vi "MICSD Zarlink Telemetry.vi"(6 "Transceive Delay mS":dbl=200.0 min=0.0 max=10000.0 step=1.0, 7 "EXID":u32=16773121 step=1 format="%.0x", 8 "Parameters":string, 9 "CP_DATA IN":u8[](array[numeric]), 10 "Function":T3(ring)=enum."Downlink Only", 11 "Command":T2) -> (0 "Data":string, 1 "CP_DATA OUT":u8[](array[numeric]), 2 "Response Code":string, 3 "Response Token":string, 4 "tChecksum Valid":bool, 5 "bChecksum Valid":bool)   [LabVIEW 2010]
uses:
  Zarlink Telemetry v9_0/Telemetry/Typedef Command List.ctl
  <vilib>/Utility/file.llb/Write To Spreadsheet File (string).vi
panel:
  out "Status Flags":T1
  in  "RF_Channel":u8=3
  in  "VISA Resource Name":refnum<visa-resource-name>="COM3"
  in  "Target MICS ID":u32=1048576 step=1 format="%.0x"
  out "error out":errorcluster
  in  "error in (no error)":errorcluster
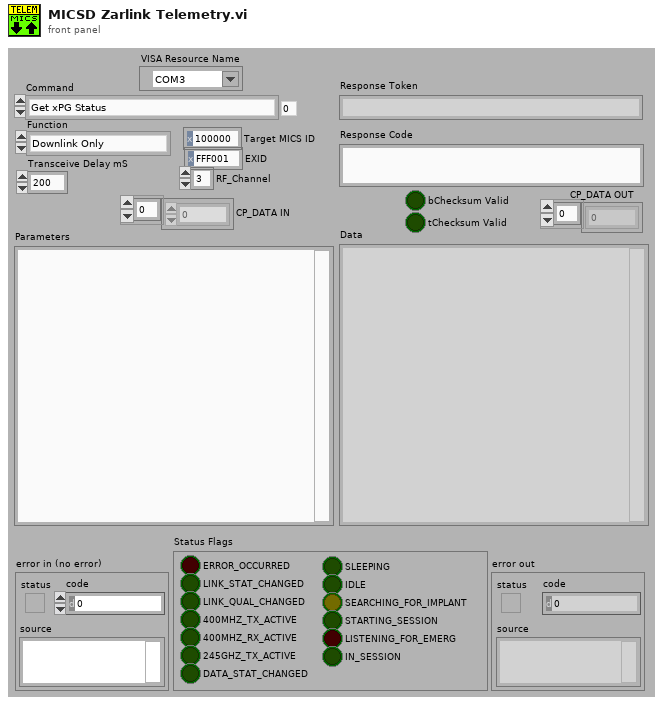
[diagram p1: front panel]
types:
  T1 = cluster{"ERROR_OCCURRED":bool, "LINK_STAT_CHANGED":bool, "LINK_QUAL_CHANGED":bool, "400MHZ_TX_ACTIVE":bool, "400MHZ_RX_ACTIVE":bool, "245GHZ_TX_ACTIVE":bool, "DATA_STAT_CHANGED":bool, "SLEEPING":bool, "IDLE":bool, "SEARCHING_FOR_IMPLANT":bool, "STARTING_SESSION":bool, "LISTENING_FOR_EMERG":bool, "IN_SESSION":bool}
  T2 = typedef "Typedef Command List.ctl" = enum16{"Get xPG Status", "xPG Stimulation", "Select Program", "Increment Program Amplitude", "Decrement Program Amplitude", "Get PoP Constants", "Get PPC Constants", "Get Program Names", "Set Pulse Amplitude", "Increment Pulse Amplitude", "Decrement Pulse Amplitude", "Get Pulse Widths", "Set Pulse Widths", "Increment Pulse Width", "Decrement Pulse Width", "Get Program Frequency", "Set Program Frequency", "Increment Program Frequency", "Decrement Program Frequency", "<reserved 1>", "Charging Control", "Get xPG Identity", "Set xPG Identity", "Restore Program Defaults", "Get Program Definition", "Set Program Definition", "Get Program Constants", "Set Program Constants", "Get Configurable Device Parameters", "Set Configurable Device Parameters", "Get Pulse Constants", "Set Pulse Constants", "Get Lead Limits", "Set Lead Limits", "Get Channel Calibrations", "Set Channel Calibrations", "<reserved 2>", "<reserved 3>", "<reserved 4>", "<reserved 5>", "<reserved 6>", "<reserved 7>", "Get Stim Asic HV Calibrations", "Set Stim Asic HV Calibrations", "<reserved 8>", "<reserved 9>", "Get CP Data", "Set CP Data", "Clear Log", "Read Log", "Append Log", "Get Patient Program Runtime", "Set Patient Program Runtime", "Impedance Measurement", "Enter Storage Mode", "Echo Short", "Echo Long", "Get General Calibration", "Set General Calibration", "Get Trim List", "Set Trim List", "Get Counter", "Set Counter", "Get Test Stimulation", "Set Test Stimulation", "Get Titration Stimulation", "Set Titration Stimulation", "Get Ramp Time", "Set Ramp Time", "Get VBAT", "Set Software Description Block", "Get Software Description Block", "Write Memory", "Read Memory", "Reset xPG", "Erase Flash Block", "Write Vectors", "Read Vectors", "Diagnostic Data", "Set Background Impedance", "Get Background Impedence ", "Undefined"}
  T3 = enum16{"Open Session", "Close Session", "Downlink Only", "Uplink Only", "Transceive (DN -> UP)"}
  T4 = cluster{"ConfigFlags":u8, "ImplantID":u32, "CompanyID":u8, "Normal_Comm":cluster{"RF_Channel":u8, "UserData":u8, "TX_Mod":u8, "RX_Mod":u8, "RX_BlockSize":u8, "BlockPerPack":u8, "TX_BlockSize":u8}, "Emerg_Comm":cluster{"RF_Channel":u8, "UserData":u8, "TX_Mod":u8, "RX_Mod":u8, "TX_BlockSize":u8, "BlockPerPack":u8, "RX_BlockSize":u8}, "ImplantRev":u8, "245TX_PowerCal":i8, "245TX_Power":i8, "CCA_RSSI_Thresholds":cluster{"ch0":u16, "ch1":u16, "ch2":u16, "ch3":u16, "ch4":u16, "ch5":u16, "ch6":u16, "ch7":u16, "ch8":u16, "ch9":u16}}
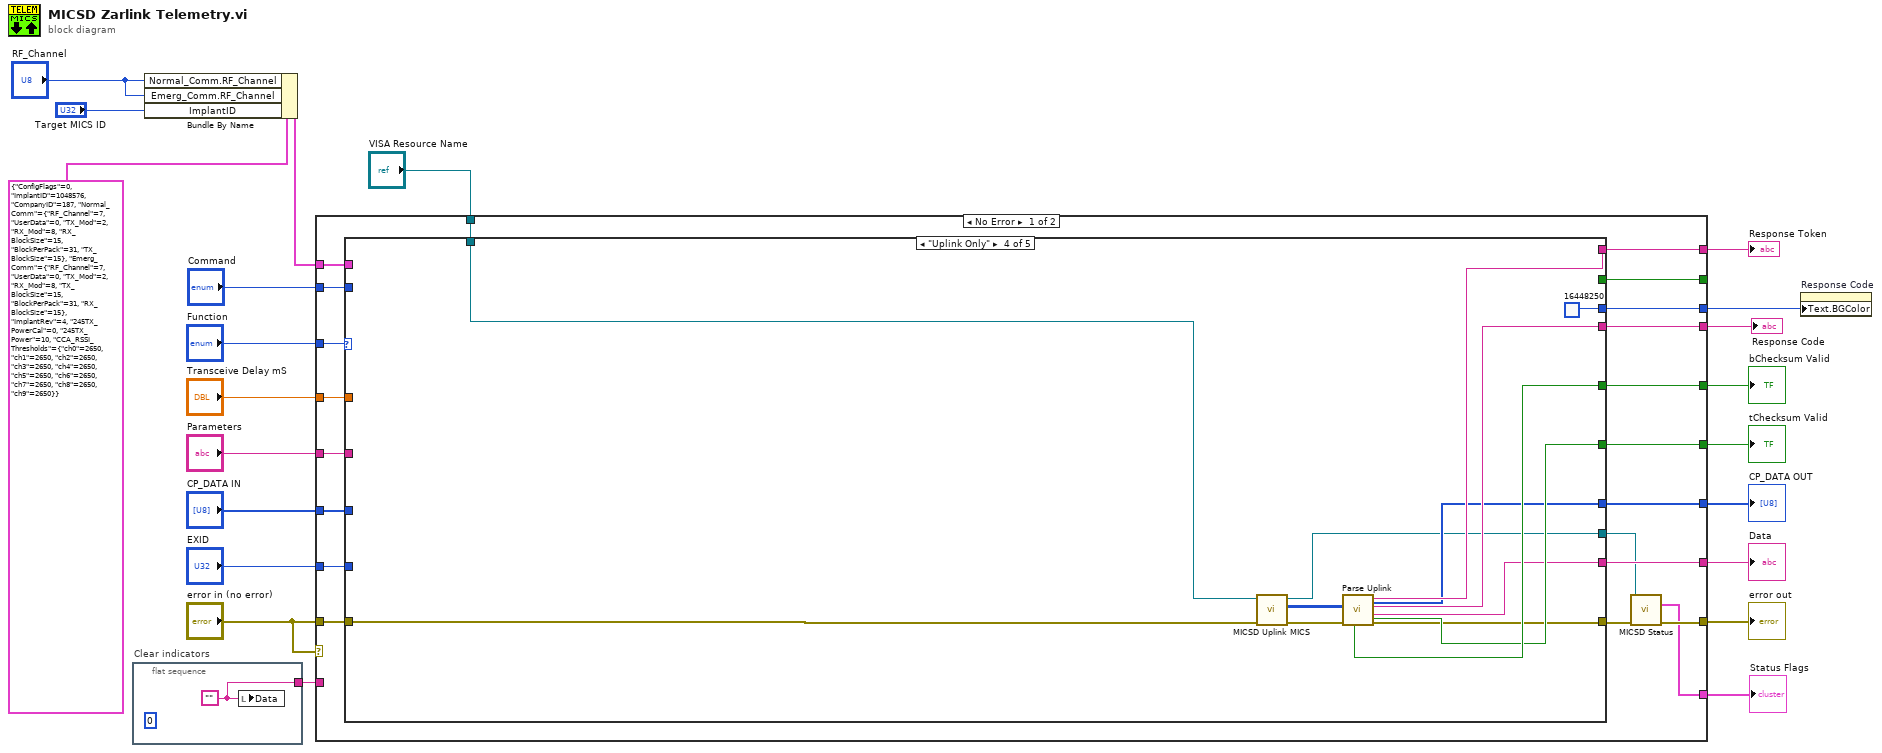
[diagram p0: block diagram]
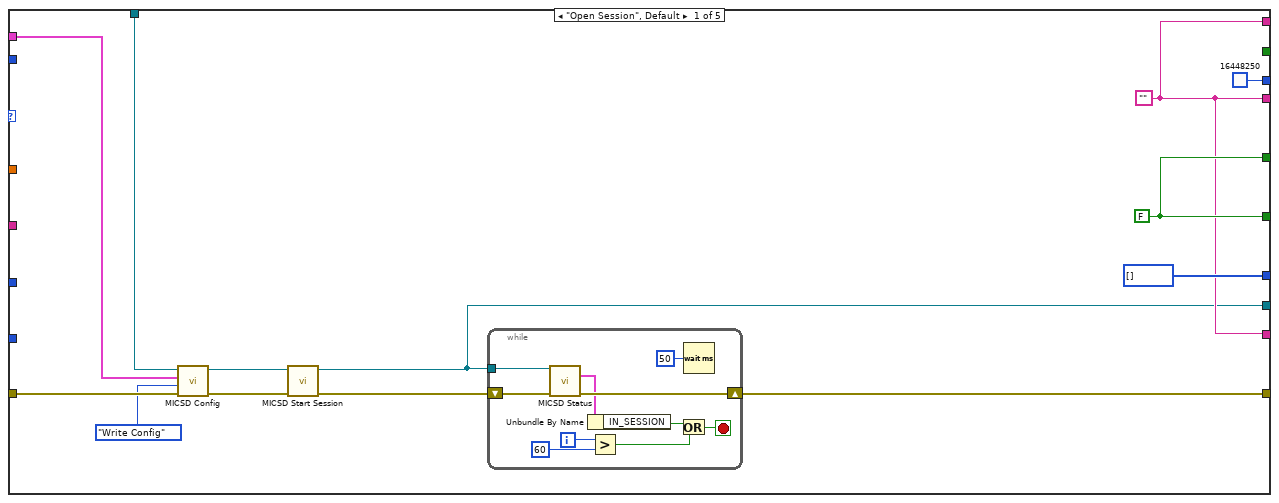
[diagram p2: hidden frame]
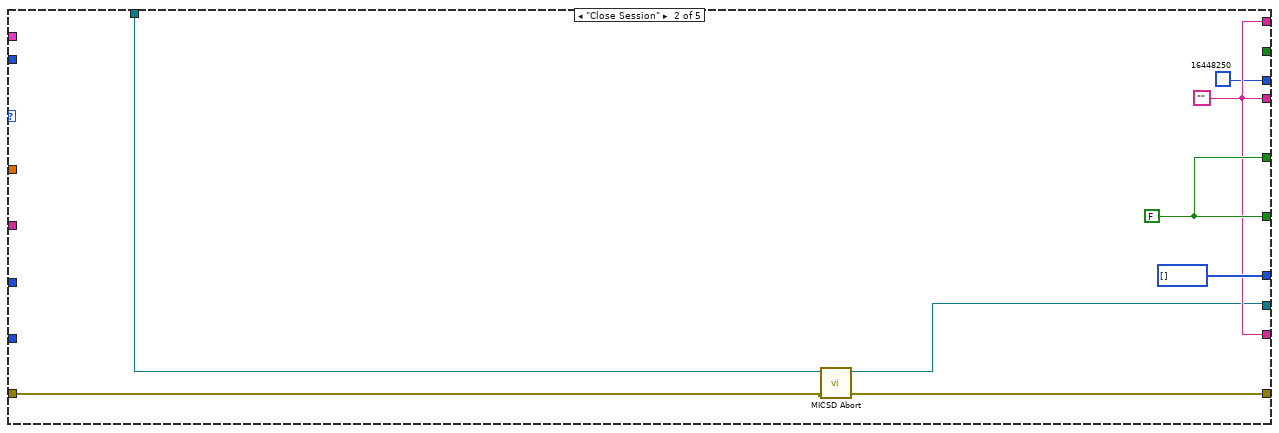
[diagram p3: hidden frame]
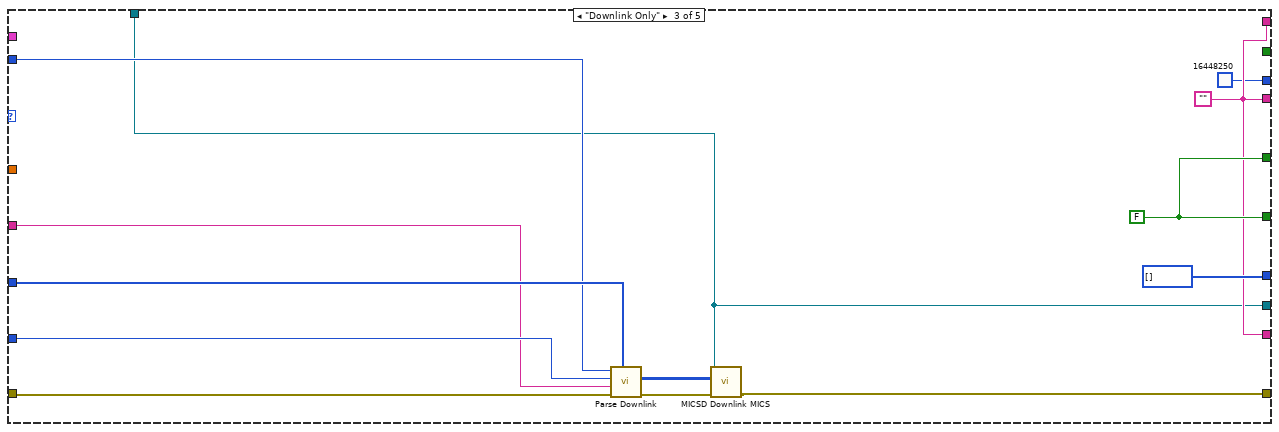
[diagram p4: hidden frame]
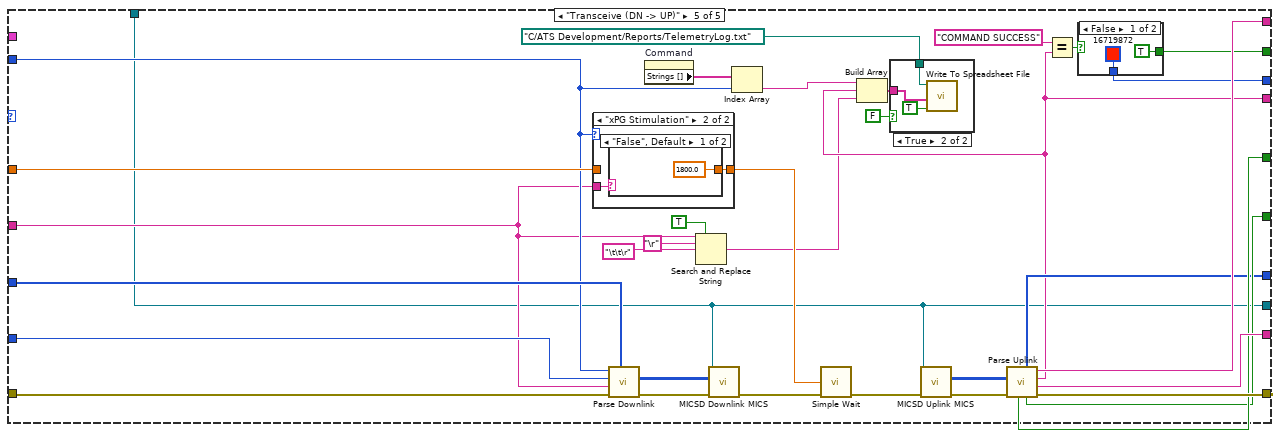
[diagram p5: hidden frame]
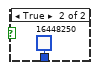
[diagram p6: hidden frame]
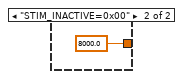
[diagram p9: hidden frame]
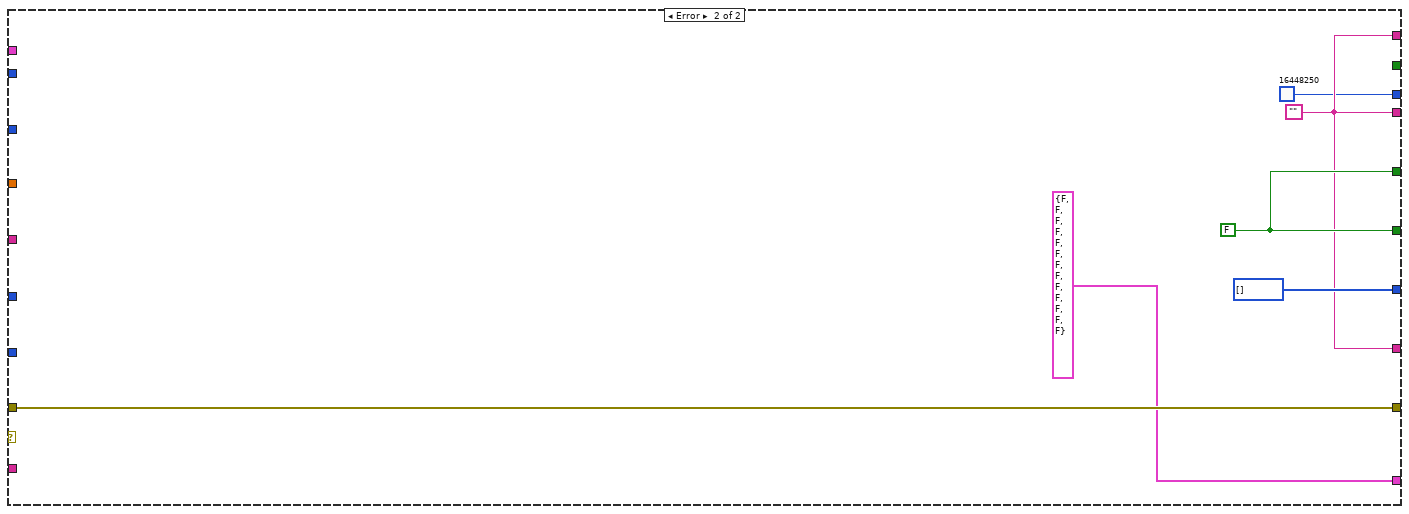
[diagram p10: hidden frame]
diagram:
  n1 = flat-sequence "Clear indicators" {
    tunnel: [w23] -> w16
    frame #0 {
      (unwired) 0 ("Connection Attempt")
      w23 = ""
      n2 = local write "Data"(w23) -> ()
    }
  }
  n3 = Bundle By Name(cluster=T4 {"ConfigFlags"=0, "ImplantID"=1048576, "CompanyID"=187, "Normal_Comm"={"RF_Channel"=7, "UserData"=0, "TX_Mod"=2, "RX_Mod"=8, "RX_BlockSize"=15, "BlockPerPack"=31, "TX_BlockSize"=15}, "Emerg_Comm"={"RF_Channel"=7, "UserData"=0, "TX_Mod"=2, "RX_Mod"=8, "TX_BlockSize"=15, "BlockPerPack"=31, "RX_BlockSize"=15}, "ImplantRev"=4, "245TX_PowerCal"=0, "245TX_Power"=10, "CCA_RSSI_Thresholds"={"ch0"=2650, "ch1"=2650, "ch2"=2650, "ch3"=2650, "ch4"=2650, "ch5"=2650, "ch6"=2650, "ch7"=2650, "ch8"=2650, "ch9"=2650}} ("MICS_Config_In"), "Normal_Comm.RF_Channel"="RF_Channel", "Emerg_Comm.RF_Channel"="RF_Channel", "ImplantID"="Target MICS ID") -> (w15:T4)
  n4 = case shown="No Error" "error in (no error)" {
    tunnel: "error in (no error)" -> [w44 w151]
    tunnel: [w26 w151] -> w13
    tunnel: "Function" -> [w43 _]
    tunnel: "Transceive Delay mS" -> [w36 _]
    tunnel: [w37 w148] -> w7
    tunnel: [w38 w148] -> w8
    tunnel: [w39 w150] -> w9
    tunnel: [w40 w150] -> w10
    tunnel: [w41 u8[] [] ("CP_DATA OUT")] -> w11
    tunnel: [w42 w148] -> w12
    tunnel: "CP_DATA IN" -> [w35 _]
    tunnel: "Command" -> [w34 _]
    tunnel: "EXID" -> [w33 _]
    tunnel: "Parameters" -> [w32 _]
    tunnel: w15 -> [w31 _]
    tunnel: w16 -> [_ _]
    tunnel: [w30 u32 16448250] -> w14
    tunnel: [w29 _] -> _
    tunnel: "VISA Resource Name" -> [w28 _]
    tunnel: [w24 T1 {"ERROR_OCCURRED"=FALSE, "LINK_STAT_CHANGED"=FALSE, "LINK_QUAL_CHANGED"=FALSE, "400MHZ_TX_ACTIVE"=FALSE, "400MHZ_RX_ACTIVE"=FALSE, "245GHZ_TX_ACTIVE"=FALSE, "DATA_STAT_CHANGED"=FALSE, "SLEEPING"=FALSE, "IDLE"=FALSE, "SEARCHING_FOR_IMPLANT"=FALSE, "STARTING_SESSION"=FALSE, "LISTENING_FOR_EMERG"=FALSE, "IN_SESSION"=FALSE} ("Status Flags")] -> w1
    frame No Error {
      n5 = case shown="\"Uplink Only\"" w43 {
        tunnel: w44 -> [w52 w70 w85 w91 w133]
        tunnel: [w46 w69 w77 w94 w129] -> w27
        tunnel: [w48 w72 w78 w95 w128] -> w42
        tunnel: [u8[] [] ("CP_DATA OUT") u8[] [] ("CP_DATA OUT") u8[] [] ("CP_DATA OUT") w96 w124] -> w41
        tunnel: [w56 w73 w80 w97 w125] -> w40
        tunnel: [w56 w73 w80 w98 w126] -> w39
        tunnel: [w48 w72 w78 w99 w113] -> w38
        tunnel: [w48 w72 w78 w100 w127] -> w37
        tunnel: w36 -> [_ _ _ _ w118]
        tunnel: w35 -> [_ _ w83 _ w132]
        tunnel: w34 -> [_ _ w81 _ w115]
        tunnel: w33 -> [_ _ w84 _ w131]
        tunnel: w32 -> [_ _ w82 _ w109]
        tunnel: w31 -> [w47 _ _ _ _]
        tunnel: [u32 16448250 u32 16448250 u32 16448250 u32 16448250 w103] -> w30
        tunnel: [_ _ _ _ w102] -> w29
        tunnel: w28 -> [w53 w68 w75 w89 w101]
        tunnel: [w45 w67 w75 w88 w101] -> w25
        frame "Open Session", Default {
          w48 = ""
          w56 = FALSE
          n6 = call "MICSD Config.vi"("error in (no error)"=w52, "Function"=enum16{"Write Config", "Read Config"}."Write Config", "MICS_Config_In"=w47, "VISA Resource Name"=w53) -> ("error out"=w50:errorcluster, "dup VISA Resource Name"=w49:refnum<visa-resource-name>)  [unwired: 5 in, 1 out]
          n7 = call "MICSD Start Session.vi"("error in (no error)"=w50, "VISA Resource Name"=w49) -> ("error out"=w46:errorcluster, "dup VISA Resource Name"=w45:refnum<visa-resource-name>)  [unwired: 8 in]
          n8 = while {
            tunnel: w45 -> [w65]
            shift-right: [w64] -> _
            shift-left: w46 -> [w66]
            i -> [w58]
            stop <- w59 stop-if-true
            n9 = call "MICSD Status.vi"("VISA Resource Name"=w65, "error in (no error)"=w66) -> ("Status Flags"=w63:T1, "error out"=w64:errorcluster)  [unwired: 7 in, 5 out]
            n10 = Unbundle By Name(w63) -> ("IN_SESSION"=w61:bool)
            n11 = Greater?(x=w58, y=60) -> (0:w60:bool)
            n12 = Or(x=w61, y=w60) -> (x .or. y?=w59:bool)
            n13 = Wait (ms)(milliseconds to wait=u32 50) -> ()  [unwired: 1 out]
          }
        }
        frame "Close Session" {
          w72 = ""
          w73 = FALSE
          n14 = call "MICSD Abort.vi"("error in (no error)"=w70, "VISA Resource Name"=w68) -> ("error out"=w69:errorcluster, "dup VISA Resource Name"=w67:refnum<visa-resource-name>)  [unwired: 8 in]
        }
        frame "Downlink Only" {
          w78 = ""
          w80 = FALSE
          n15 = call "Parse Downlink.vi"("CP_DATA IN"=w83, "error in (no error)"=w85, "Parameters"=w82, "EXID"=w84, "Command"=w81) -> ("error out"=w87:errorcluster, "Downlink"=w86:u8[][])  [unwired: 5 in]
          n16 = call "MICSD Downlink MICS.vi"("Error In"=w87, "Downlink"=w86, "VISA Resource Name"=w75) -> ("Error Out"=w77:errorcluster)  [unwired: 7 in, 1 out]
        }
        frame "Uplink Only" {
          n17 = call "MICSD Uplink MICS.vi"("Error In"=w91, "VISA Resource Name"=w89) -> ("Error Out"=w92:errorcluster, "Uplink"=w90:u8[][], "dup VISA Resource Name"=w88:refnum<visa-resource-name>)  [unwired: 7 in]
          n18 = call "Parse Uplink.vi"("error in (no error)"=w92, "Uplink"=w90) -> ("error out"=w94:errorcluster, "Data"=w95:string, "Response Code"=w99:string, "Response Token"=w100:string, "tChecksum Valid"=w97:bool, "CP_DATA"=w96:u8[], "bChecksum Valid"=w98:bool)  [unwired: 3 in]
        }
        frame "Transceive (DN -> UP)" {
          n19 = case shown="\"xPG Stimulation\"" w115 {
            tunnel: w118 -> [w141 _]
            tunnel: [w141 w142] -> w117
            tunnel: w109 -> [_ w143]
            frame "Get xPG Status", Default {
            }
            frame "xPG Stimulation" {
              n20 = case shown="\"False\", Default" w143 {
                tunnel: [1800.0 ("Transceive Delay mS") 8000.0 ("Transceive Delay mS")] -> w142
                frame "False", Default {
                }
                frame "STIM_INACTIVE=0x00" {
                }
              }
            }
          }
          n21 = call "Parse Downlink.vi"("CP_DATA IN"=w132, "error in (no error)"=w133, "Parameters"=w109, "EXID"=w131, "Command"=w115) -> ("error out"=w134:errorcluster, "Downlink"=w122:u8[][])  [unwired: 5 in]
          n22 = property on="Command" class="Enum (strict)"() -> ("Strings []"=w116:string[])  [unwired: 2 in, 2 out]
          n23 = Search and Replace String(replace all?=TRUE ("replace all? (F)"), input string=w109, search string="\r", replace string="\t\t\r" ("search string")) -> (result string=w110:string)  [unwired: 4 in, 3 out]
          n24 = call "MICSD Downlink MICS.vi"("Error In"=w134, "Downlink"=w122, "VISA Resource Name"=w101) -> ("Error Out"=w121:errorcluster)  [unwired: 7 in, 1 out]
          n25 = Index Array(array=w116, index=w115) -> (element=w114:string)
          n26 = call "Simple Wait.vi"("mS"=w117, "error in"=w121) -> ("error out"=w120:errorcluster)  [unwired: 12 in, 1 out]
          n27 = call "MICSD Uplink MICS.vi"("Error In"=w120, "VISA Resource Name"=w101) -> ("Error Out"=w130:errorcluster, "Uplink"=w123:u8[][])  [unwired: 7 in, 1 out]
          n28 = call "Parse Uplink.vi"("error in (no error)"=w130, "Uplink"=w123) -> ("error out"=w129:errorcluster, "Data"=w128:string, "Response Code"=w113:string, "Response Token"=w127:string, "tChecksum Valid"=w125:bool, "CP_DATA"=w124:u8[], "bChecksum Valid"=w126:bool)  [unwired: 3 in]
          n29 = Build Array(w114, w113, w110) -> (w111:string[])
          n30 = case shown="True" FALSE {
            tunnel: path "C:/ATS Development/Reports/TelemetryLog.txt" ("file (use dialog)") -> [_ w140]
            tunnel: w111 -> [_ w139]
            frame False {
            }
            frame True {
              n31 = call-poly <vilib>:"Write To Spreadsheet File.vi"("append to file? (new file:F)"=TRUE, "1D data"=w139, "file path (dialog if empty)"=w140) -> ()  [unwired: 5 in, 1 out]
            }
          }
          n32 = Equal?(x="COMMAND SUCCESS", y=w113) -> (x = y?=w104:bool)
          n33 = case shown="False" w104 {
            tunnel: [u32 16719872 u32 16448250] -> w103
            tunnel: [TRUE _] -> w102
            frame False {
            }
            frame True {
            }
          }
        }
      }
      n34 = call "MICSD Status.vi"("VISA Resource Name"=w25, "error in (no error)"=w27) -> ("Status Flags"=w24:T1, "error out"=w26:errorcluster)  [unwired: 7 in, 5 out]
    }
    frame Error {
      w148 = ""
      w150 = FALSE
    }
  }
  "error out" <- w13
  "Response Token" <- w7
  "Response Code" <- w8
  "Data" <- w12
  "CP_DATA OUT" <- w11
  "tChecksum Valid" <- w10
  "bChecksum Valid" <- w9
  "Status Flags" <- w1
  n35 = property on="Response Code" class="Str"("Text.BGColor"=w14) -> ()  [unwired: 2 in, 2 out]
